vi "Controller Extract FOFB Variables.vi"(0 "FOFB Configuration":T1, 1 "Selected Reference Orbit":i32, 2 "Selected Correction Matrix":i32, 3 "Selected FPGA Filters":i32, 11 "error in (no error)":errorcluster) -> (4 "FOFB Variables":T7, 15 "error out":errorcluster)   [LabVIEW 2011, in "Controller VIs.lvlib"]
uses:
  Controller VIs.lvlib
  Types Definitions/Type FOFB Variables.ctl
  Types Definitions/Type FOFB Configuration.ctl
  Types Definitions/Type FOFB Parameters.ctl
  Types Definitions/Type Network Configuration.ctl
  Types Definitions/Type FA Configuration.ctl
  Types Definitions/Type Acquisition Network Configuration.ctl
  Types Definitions/Type Actuation Network Configuration.ctl
  Type Definitions.lvlib
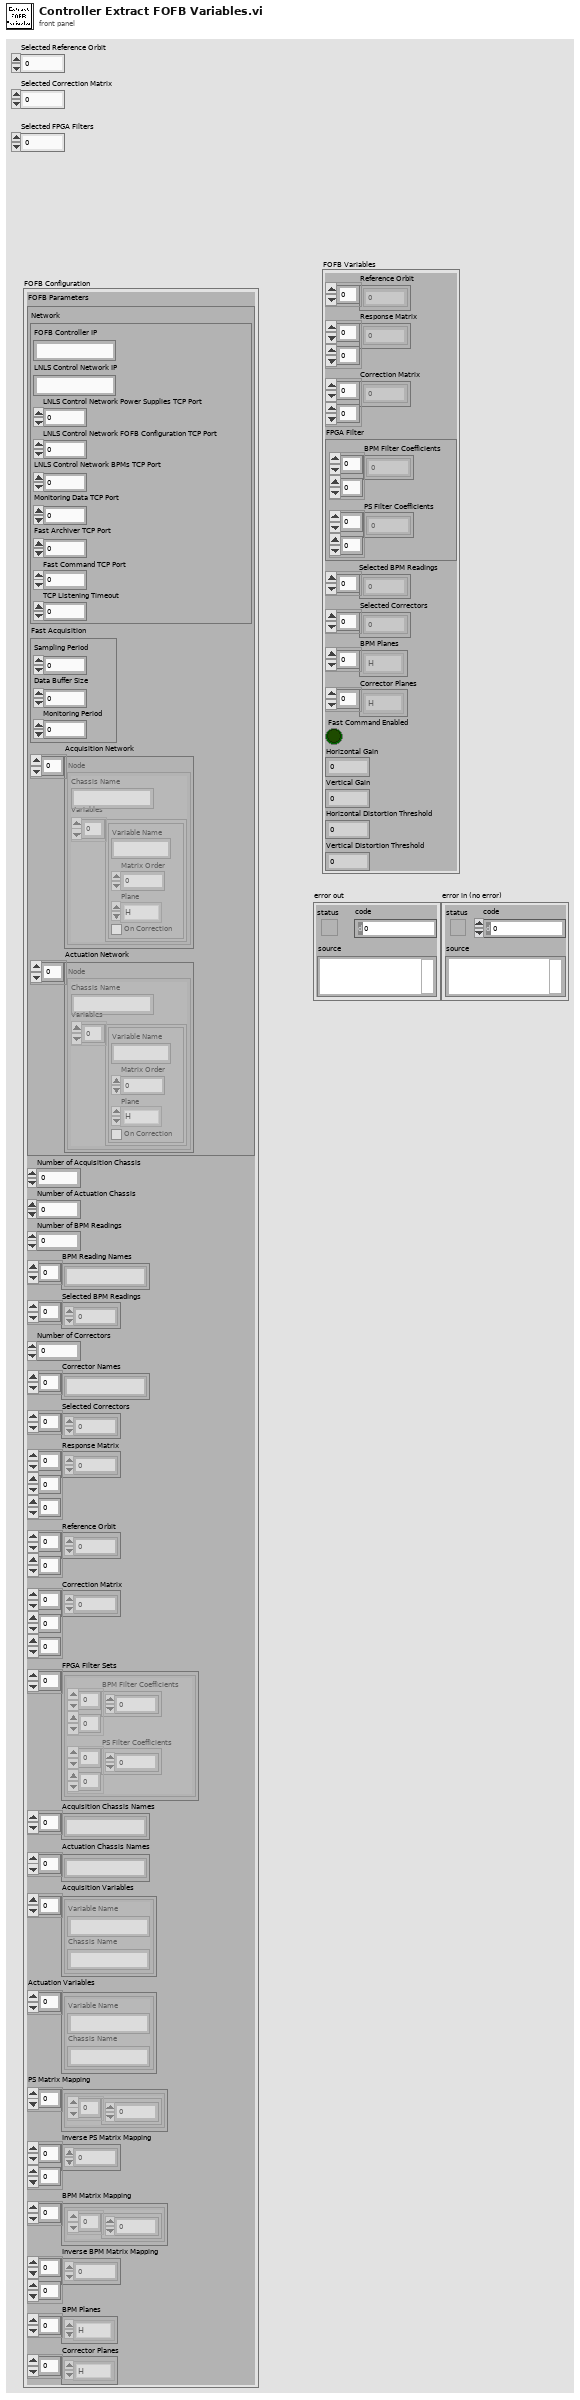
[diagram p1: front panel]
types:
  T1 = typedef "Type Definitions.lvlib/Type FOFB Configuration.ctl" = cluster{"FOFB Parameters":T2, "Number of Acquisition Chassis":i32, "Number of Actuation Chassis":i32, "Number of BPM Readings":i32, "BPM Reading Names":string[], "Selected BPM Readings":u32[], "Number of Correctors":i32, "Corrector Names":string[], "Selected Correctors":u32[], "Response Matrix":dbl[][][], "Reference Orbit":dbl[][], "Correction Matrix":dbl[][][], "FPGA Filter Sets":cluster{"BPM Filter Coefficients":dbl[][], "PS Filter Coefficients":dbl[][]}[], "Acquisition Chassis Names":string[], "Actuation Chassis Names":string[], "Acquisition Variables":cluster{"Variable Name":string, "Chassis Name":string}[], "Actuation Variables":cluster{"Variable Name":string, "Chassis Name":string}[], "PS Matrix Mapping":cluster{u32[]}[], "Inverse PS Matrix Mapping":u32[][], "BPM Matrix Mapping":cluster{u32[]}[], "Inverse BPM Matrix Mapping":u32[][], "BPM Planes":enum8{"H", "V"}[], "Corrector Planes":enum8{"H", "V"}[]}
  T2 = typedef "Type Definitions.lvlib/Type FOFB Parameters.ctl" = cluster{"Network":T3, "Fast Acquisition":T4, "Acquisition Network":T5, "Actuation Network":T6}
  T3 = typedef "Type Definitions.lvlib/Type Network Configuration.ctl" = cluster{"FOFB Controller IP":string, "LNLS Control Network IP":string, "LNLS Control Network Power Supplies TCP Port":u16, "LNLS Control Network FOFB Configuration TCP Port":u16, "LNLS Control Network BPMs TCP Port":u16, "Monitoring Data TCP Port":u16, "Fast Archiver TCP Port":u16, "Fast Command TCP Port":u16, "TCP Listening Timeout":i32}
  T4 = typedef "Type Definitions.lvlib/Type FA Configuration.ctl" = cluster{"Sampling Period":u32, "Data Buffer Size":u32, "Monitoring Period":u32}
  T5 = typedef "Type Definitions.lvlib/Type Acquisition Network Configuration.ctl" = cluster{"Chassis Name":string, "Variables":cluster{"Variable Name":string, "Matrix Order":u32, "Plane":enum8{"H", "V"}, "On Correction":bool}[]}[]
  T6 = typedef "Type Definitions.lvlib/Type Actuation Network Configuration.ctl" = cluster{"Chassis Name":string, "Variables":cluster{"Variable Name":string, "Matrix Order":u32, "Plane":enum8{"H", "V"}, "On Correction":bool}[]}[]
  T7 = typedef "Type Definitions.lvlib/Type FOFB Variables.ctl" = cluster{"Reference Orbit":dbl[], "Response Matrix":dbl[][], "Correction Matrix":dbl[][], "FPGA Filter":cluster{"BPM Filter Coefficients":dbl[][], "PS Filter Coefficients":dbl[][]}, "Selected BPM Readings":u32[], "Selected Correctors":u32[], "BPM Planes":enum8{"H", "V"}[], "Corrector Planes":enum8{"H", "V"}[], "Fast Command Enabled":bool, "Horizontal Gain":dbl, "Vertical Gain":dbl, "Horizontal Distortion Threshold":dbl, "Vertical Distortion Threshold":dbl}
  T8 = cluster{"BPM Filter Coefficients":dbl[][], "PS Filter Coefficients":dbl[][]}[]
  T9 = cluster{"BPM Filter Coefficients":dbl[][], "PS Filter Coefficients":dbl[][]}
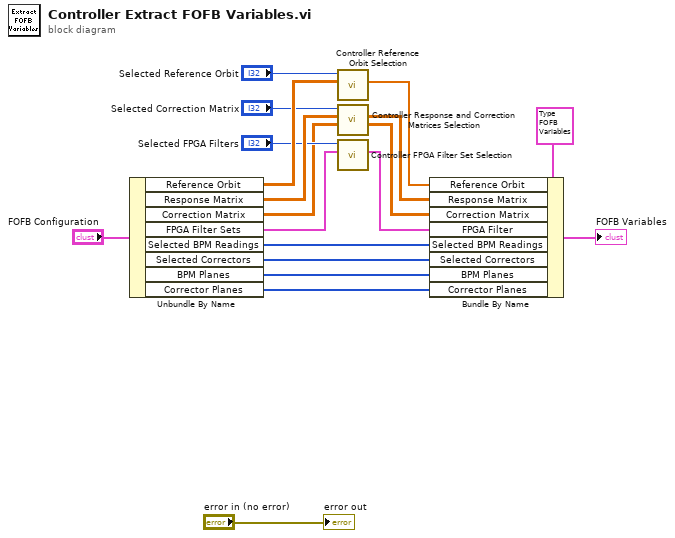
[diagram p0: block diagram]
diagram:
  n1 = Unbundle By Name("FOFB Configuration") -> ("Reference Orbit"=w11:dbl[][], "Response Matrix"=w8:dbl[][][], "Correction Matrix"=w4:dbl[][][], "FPGA Filter Sets"=w7:T8, "Selected BPM Readings"=w17:u32[], "Selected Correctors"=w16:u32[], "BPM Planes"=w15:enum8{"H", "V"}[], "Corrector Planes"=w14:enum8{"H", "V"}[])
  n2 = call "Controller Reference Orbit Selection.vi"("Reference Orbits"=w11, "selected"="Selected Reference Orbit") -> ("Selected Reference Orbit"=w1:dbl[])  [unwired: 9 in]
  n3 = call "Controller Response and Correction Matrices Selection.vi"("Correction  Matrices"=w4, "Response Matrices"=w8, "selected"="Selected Correction Matrix") -> ("Selected Correction Matrix"=w3:dbl[][], "Selected Response Matrix"=w2:dbl[][])  [unwired: 7 in]
  n4 = call "Controller FPGA Filter Set Selection.vi"("FPGA Filter Sets"=w7, "selected"="Selected FPGA Filters") -> ("Selected FPGA Filter Set"=w5:T9)  [unwired: 9 in]
  n5 = Bundle By Name(cluster=T7 {"Reference Orbit"=[], "Response Matrix"=[], "Correction Matrix"=[], "FPGA Filter"={"BPM Filter Coefficients"=[], "PS Filter Coefficients"=[]}, "Selected BPM Readings"=[], "Selected Correctors"=[], "BPM Planes"=[], "Corrector Planes"=[], "Fast Command Enabled"=FALSE, "Horizontal Gain"=0.0, "Vertical Gain"=0.0, "Horizontal Distortion Threshold"=0.0, "Vertical Distortion Threshold"=0.0} ("FOFB Variables 2"), "Reference Orbit"=w1, "Response Matrix"=w2, "Correction Matrix"=w3, "FPGA Filter"=w5, "Selected BPM Readings"=w17, "Selected Correctors"=w16, "BPM Planes"=w15, "Corrector Planes"=w14) -> (→"FOFB Variables":T7)
  "error out" <- "error in (no error)"
